vi "manipulator Controller.vi"(8 "error in":errorcluster) -> ()   [LabVIEW 2020]
doc: "This VI executes continuously carrying out the current operation and responding to updates or new operations. It will often contain the timing or control code that is difficult to place directly in TeleOp. This VI generally opens all sensors and motors and isolates the rest of the robot code from knowing how the operations are carried out."
uses:
  <vilib>/Rock Robotics/WPI/Framework/Completion Status.ctl
  manipulator Setpoints.ctl
  manipulator Operations.ctl
  Typedefs/Teleop Manipulator Commands.ctl
  Typedefs/Cube Shooting Presets.ctl
  <vilib>/Rock Robotics/WPI/ThirdParty/REV Robotics/REVLib/Typedef/Spark MAX Sensor Type.ctl
  <vilib>/Rock Robotics/WPI/ThirdParty/REV Robotics/REVLib/Typedef/Spark MAX Idle Mode.ctl
  <vilib>/Rock Robotics/WPI/ThirdParty/REV Robotics/REVLib/Typedef/Spark MAX Control Type.ctl
  Typedefs/Shoot Cube State.ctl
  782eae61-a325-4965-976c-c64f6a44d010.vi
  Framework/Robot Global Data.vi
  <vilib>/Rock Robotics/Network Tables/NT Write Boolean.vi
  <vilib>/ptbypt/NI_PtbyPt.lvlib
panel:
  out "Waveform Chart":cluster{u32, "mean":dbl}(graph)
  out "Abs Wrist Position":dbl
  in  "Interactive Values":T1={"Operation"=enum."Reserve", "Immediate Parameters"={"Wrist Power"=0.0, "Cascade Power"=0.0}, "Griddy Parameters"={"Griddy Command"=enum."idle", "Flip Wrist?"=FALSE}, "Reset Parameters"={"Reset Wrist"=FALSE, "Reset Cascade"=FALSE}, "Shoot Cube Parameters"={"Shot Preset"=enum."shoot mid"}}
  out "Current\nCmd":string
  in  "Buttons":cluster{"Execute Cmd":bool, "Abort Cmd":bool}
  out "Command Timing":cluster{"Start Time (ms)":u32, "Iterations":i32}
  out "Status":T5
  # "Tip: It may be helpful to observe inputs and sensor values.\nYou may also want to display tuning or debugging controls."
  # "Interactive Command: You may fill in the settings for a command\nand schedule it with the Execute button. You can observe and abort\nany command while fine tuning the code for the controller."
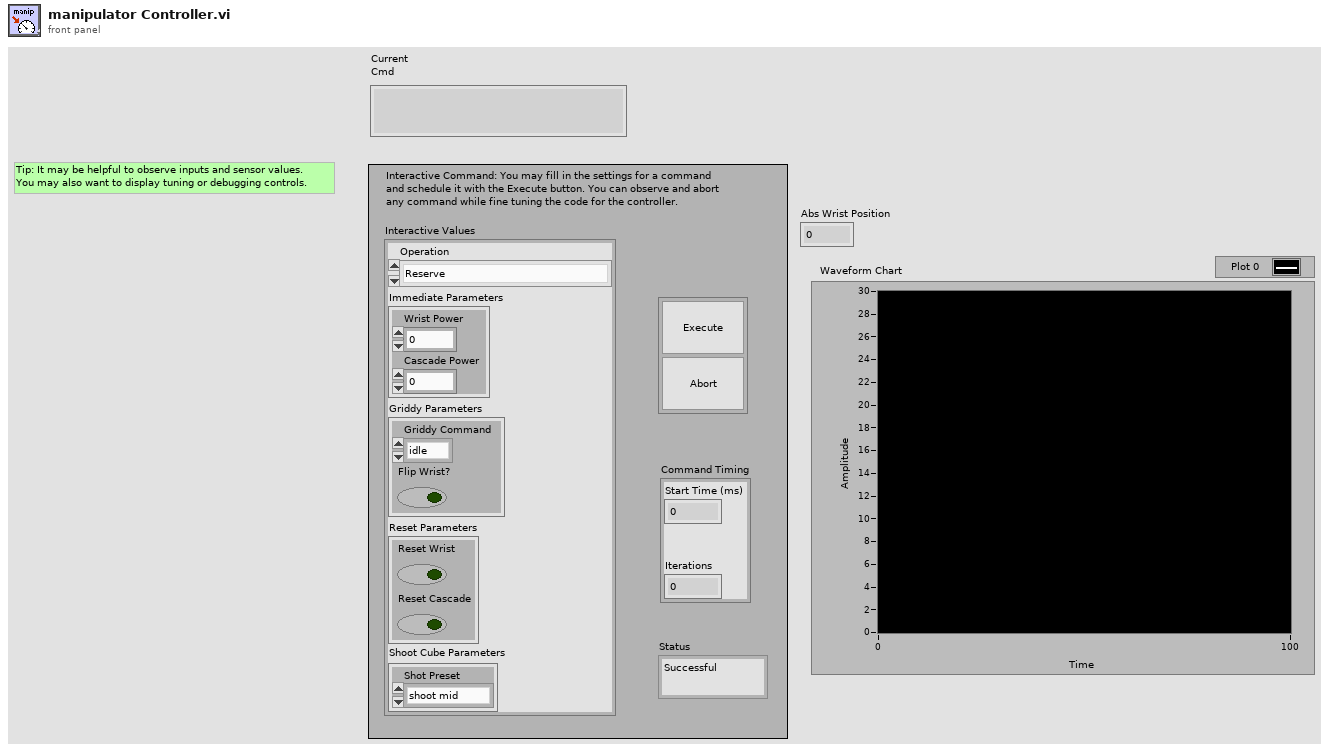
[diagram p1: front panel]
types:
  T1 = typedef "manipulator Setpoints.ctl" = cluster{"Operation":T2, "Immediate Parameters":cluster{"Wrist Power":dbl, "Cascade Power":dbl}, "Griddy Parameters":cluster{"Griddy Command":T3, "Flip Wrist?":bool}, "Reset Parameters":cluster{"Reset Wrist":bool, "Reset Cascade":bool}, "Shoot Cube Parameters":cluster{"Shot Preset":T4}}
  T2 = typedef "manipulator Operations.ctl" = enum16{"Reserve", "Read Current", "Immediate", "Reset Manipulator", "Grid-dy", "Shoot Cubes"}
  T3 = typedef "Teleop Manipulator Commands.ctl" = enum16{"idle", "intake cone sideways", "intake cone upright", "intake cone feeder", "intake cube feeder", "intake cube", "score low cone", "score low cube", "score mid cone", "score mid cube", "score high cone", "score high cube", "score mid cone up"}
  T4 = typedef "Cube Shooting Presets.ctl" = enum16{"shoot low", "shoot mid", "shoot high"}
  T5 = typedef "Completion Status.ctl" = enum16{"Successful", "Aborted", "Incomplete"}
  T6 = cluster{"P Gain":dbl, "I Gain":dbl, "D Gain":dbl, "F Gain":dbl, "I Zone":dbl, "Min Output":dbl, "Max Output":dbl}
  T7 = typedef "Spark MAX Idle Mode.ctl" = enum16{"Coast", "Brake"}
  T8 = typedef "Spark MAX Sensor Type.ctl" = enum16{"No Sensor", "Hall Sensor", "Encoder", "-Not Available-", "Analog", "Alternate Encoder", "Duty Cycle"}
  T9 = typedef "WPI_MotorControlDeviceRef.ctl" = cluster{"DeviceStatus":errorcluster, "Type":T10, "PWM":cluster{"PWM Channel":T11, "DeadBand":T12}, "CAN":cluster{"Device Number":u8, "SetOutput VI Ref":variant, "GetOutput VI Ref":variant, "Enable VI Ref":variant, "Disable VI Ref":variant, "Data":variant}, "Invert":bool, "DIO PWM":cluster{"PWM \"Enable\" Channel":T11, "DIOChannel":T13, "PWM Rate":dbl}}
  T10 = typedef "WPI_MotorControlType.ctl" = enum16{"PWM", "CAN", "DIO PWM"}
  T11 = typedef "FPGA_DIOPWMChannel.ctl" = enum8{"PWM 0", "PWM 1", "PWM 2", "PWM 3", "PWM 4", "PWM 5", "PWM 6", "PWM 7", "PWM 8", "PWM 9", "PWM MXP 0", "PWM MXP 1", "PWM MXP 2", "PWM MXP 3", "PWM MXP 4", "PWM MXP 5", "PWM MXP 6", "PWM MXP 7", "PWM MXP 8", "PWM MXP 9", "Invalid"}
  T12 = typedef "WPI_PWMDeadband.ctl" = cluster{"Name":string, "maxPositivePwm":i32, "minPositivePwm":i32, "centerPwm":i32, "maxNegativePwm":i32, "minNegativePwm":i32, "angularRange":u16}
  T13 = typedef "FPGA_DIOChannel.ctl" = enum8{"DIO 0", "DIO 1", "DIO 2", "DIO 3", "DIO 4", "DIO 5", "DIO 6", "DIO 7", "DIO 8", "DIO 9", "DIO MXP 0", "DIO MXP 1", "DIO MXP 2", "DIO MXP 3", "DIO MXP 4", "DIO MXP 5", "DIO MXP 6", "DIO MXP 7", "DIO MXP 8", "DIO MXP 9", "DIO MXP 10", "DIO MXP 11", "DIO MXP 12", "DIO MXP 13", "DIO MXP 14", "DIO MXP 15", "SPI Port CS1", "SPI Port CS2", "SPI Port CS3", "SPI Port MISO", "SPI Port MOSI", "Invalid"}
  T14 = typedef "Command Status Info.ctl" = cluster{"Name":string, "Status":T5, "notifier out":T15}
  T15 = typedef "Completion Notifier.ctl" = refnum<notifier>
  T16 = cluster{"Current Command":T1, "Command Timing":cluster{"Start Time (ms)":u32, "Iterations":i32}, "Command Arguments":cluster{"Command Info":T14, "Description":string, "Default Command":T1, "queue out":refnum<queue>, "Subsystem Name":string}}
  T17 = cluster{u32, "Immediate Parameters":cluster{"Wrist Power":dbl, "Cascade Power":dbl}}
  T18 = typedef "Spark MAX Control Type.ctl" = enum16{"Percent VBus", "Voltage", "Velocity", "Position", "Smart Motion", "Current", "Smart Velocity"}
  T19 = cluster{"Reset Wrist":bool, "Reset Cascade":bool}
  T20 = cluster{"Shot Config":cluster{"Wrist Prep Position":dbl, "Wrist Prep Margin":dbl, "Cascade Safety Position":dbl}, "Shot Parameters":cluster{"Shot Name":string, "Cascade Pow":dbl, "Shoot Position":dbl}[]}
  T21 = typedef "Shoot Cube State.ctl" = enum16{"Wrist Prep", "Shoot Cube", "Idle", "Finished"}
  T22 = cluster{"Wrist Prep Position":dbl, "Wrist Prep Margin":dbl, "Cascade Safety Position":dbl}
  T23 = cluster{"Shot Name":string, "Cascade Pow":dbl, "Shoot Position":dbl}[]
  T24 = cluster{"Shot Name":string, "Cascade Pow":dbl, "Shoot Position":dbl}
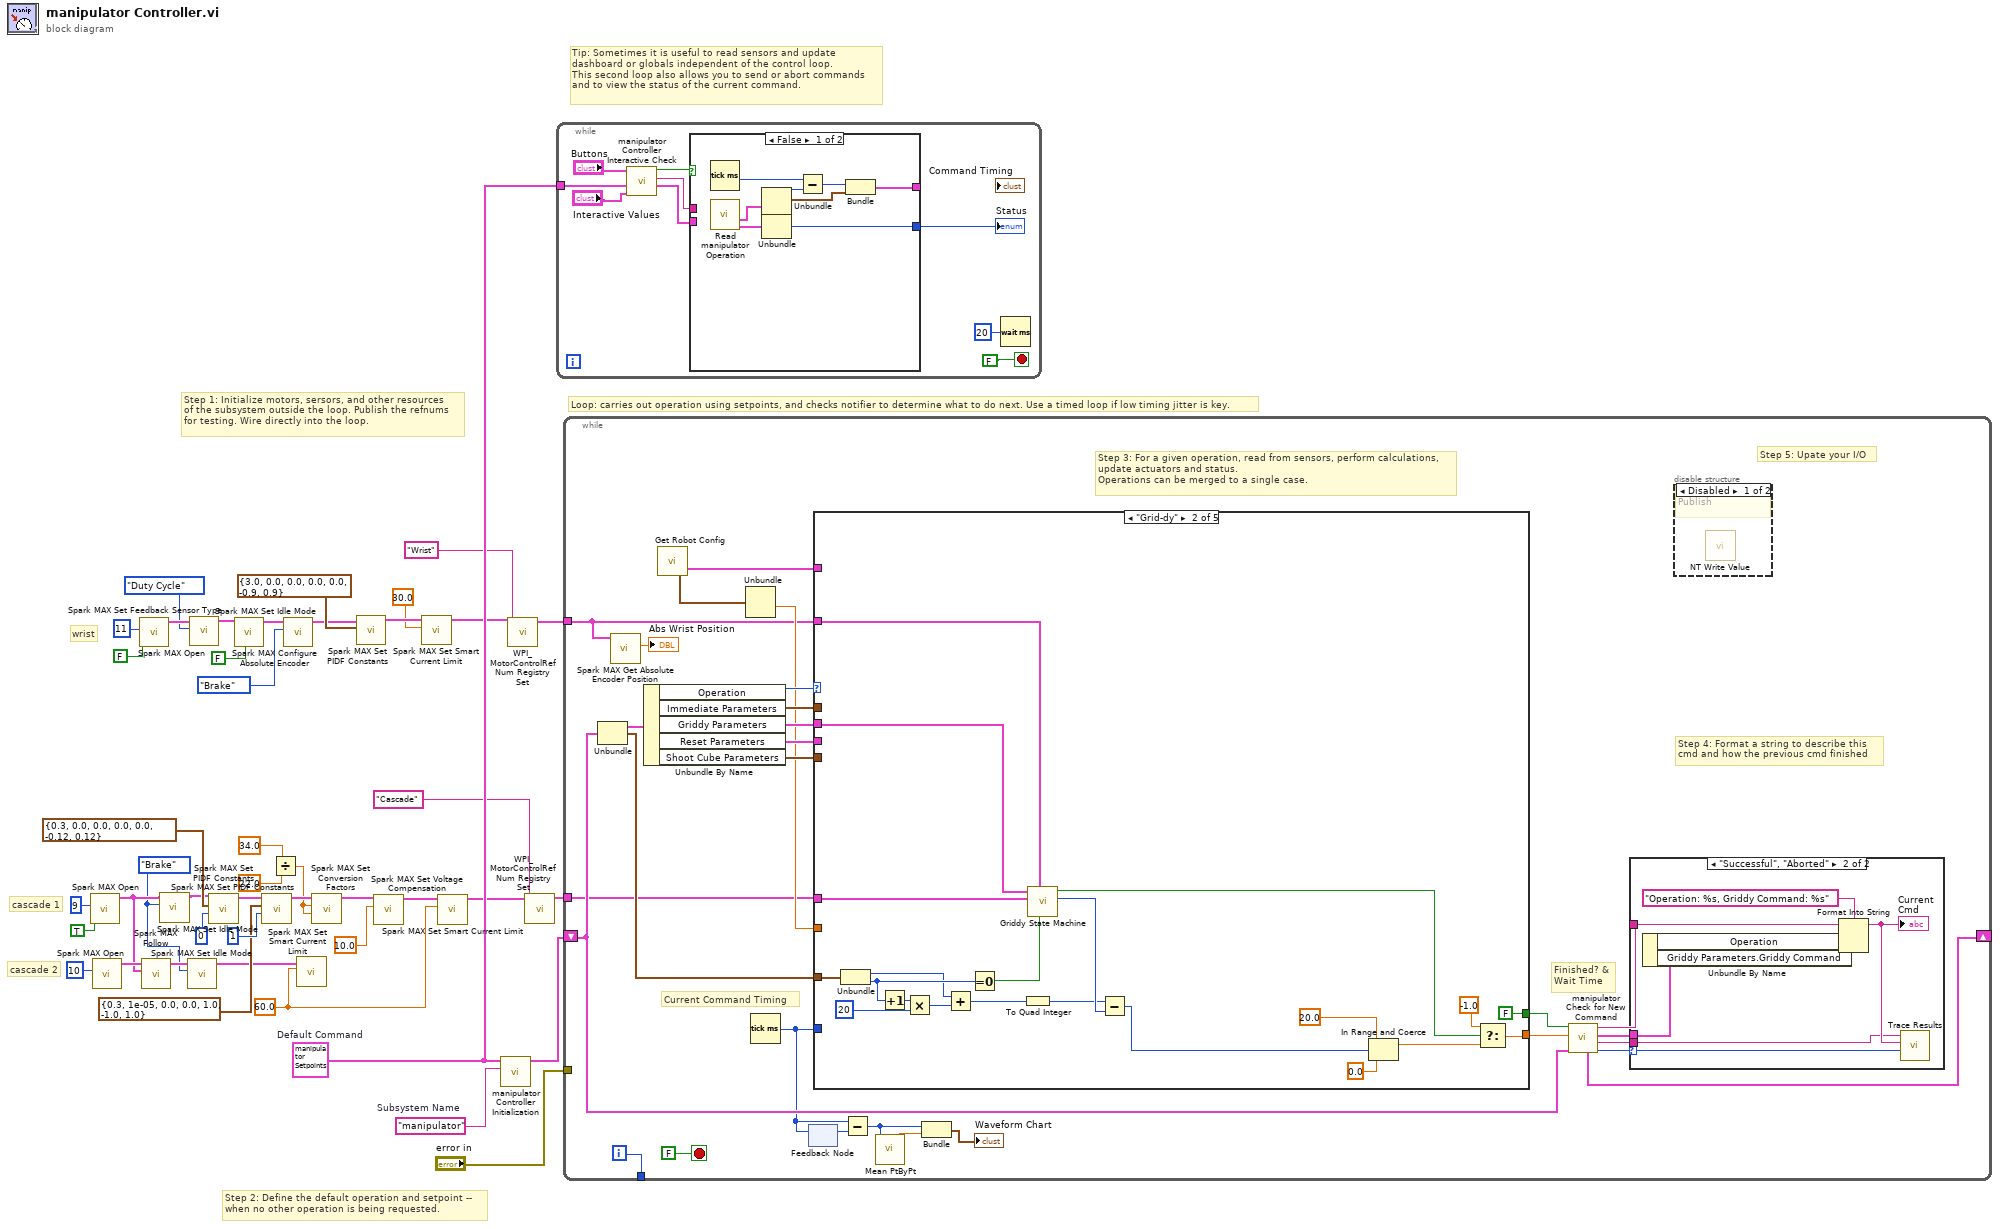
[diagram p0: block diagram]
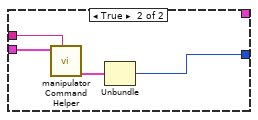
[diagram p2: hidden frame]
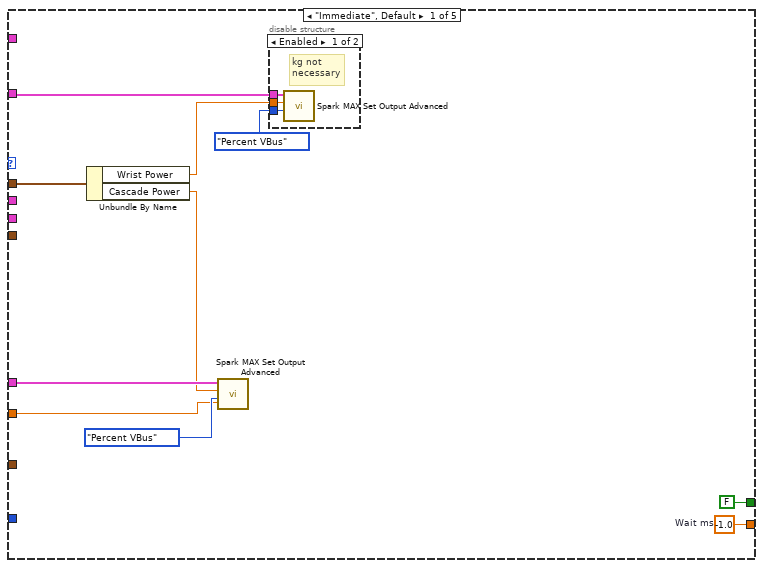
[diagram p3: hidden frame]
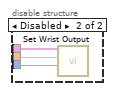
[diagram p4: hidden frame]
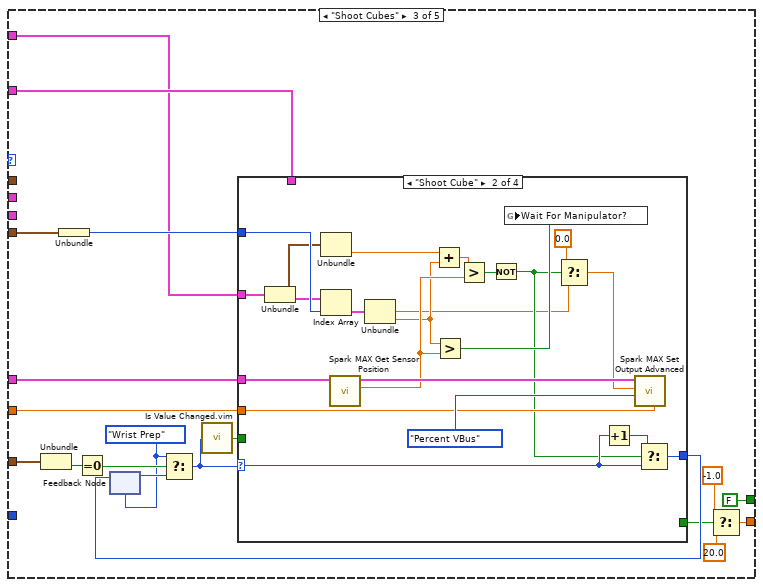
[diagram p5: hidden frame]
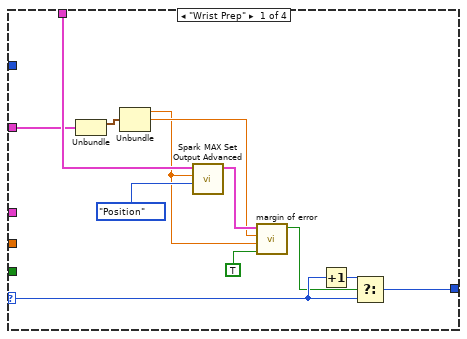
[diagram p6: hidden frame]
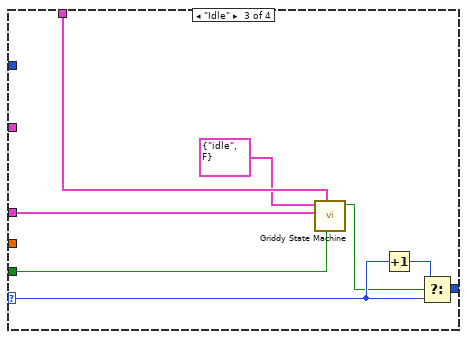
[diagram p7: hidden frame]
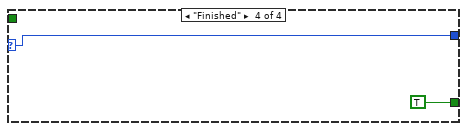
[diagram p8: hidden frame]
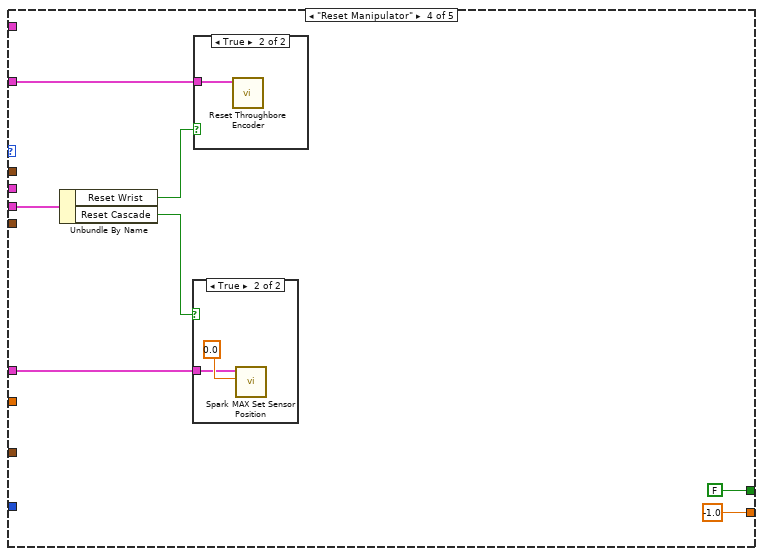
[diagram p9: hidden frame]
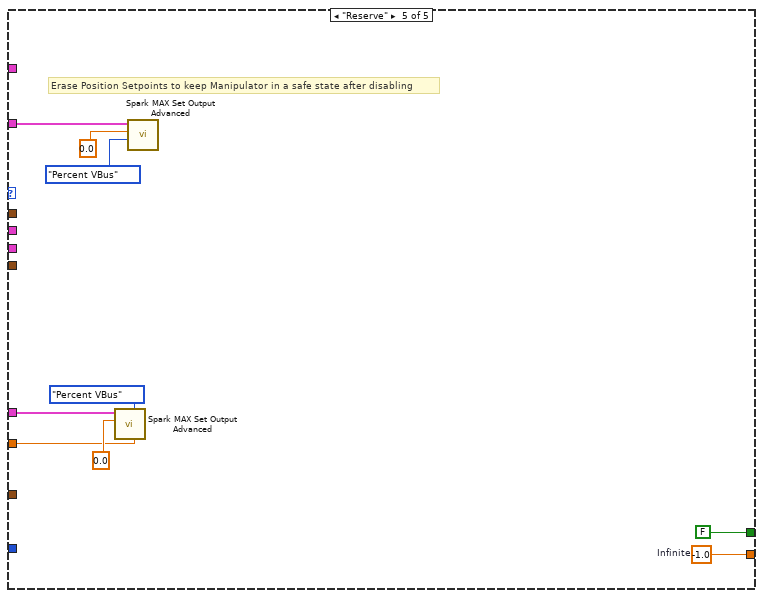
[diagram p12: hidden frame]
diagram:
  w1 = 60.0 ("Primay Current Limit (80A)")
  w15 = Spark_MAX_Idle_Mode."Brake" ("Idle Mode")
  w41 = T1 {"Operation"=enum."Reserve", "Immediate Parameters"={"Wrist Power"=0.0, "Cascade Power"=0.0}, "Griddy Parameters"={"Griddy Command"=enum."idle", "Flip Wrist?"=FALSE}, "Reset Parameters"={"Reset Wrist"=FALSE, "Reset Cascade"=FALSE}, "Shoot Cube Parameters"={"Shot Preset"=enum."shoot mid"}}  # Default Command
  w42 = "manipulator"  # Subsystem Name
  # "cascade 1"
  # "cascade 2"
  # "wrist"
  # "Tip: Sometimes it is useful to read sensors and update\ndashboard or globals independent of the control loop.\nThis second loop also allows you to send or abort commands\nand to view the status of the current command."
  # "Step 2: Define the default operation and setpoint --\nwhen no other operation is being requested."
  # "Step 1: Initialize motors, sersors, and other resources\nof the subsystem outside the loop. Publish the refnums\nfor testing. Wire directly into the loop."
  # "Loop: carries out operation using setpoints, and checks notifier to determine what to do next. Use a timed loop if low timing jitter is key."
  n1 = call <vilib>:"Spark MAX Open.vi"("Invert"=TRUE, "Device Number"=u8 9) -> ("MotorControlDeviceRef"=w35:T9)  [unwired: 8 in, 1 out]
  n2 = call <vilib>:"Spark MAX Open.vi"("Device Number"=u8 10) -> ("MotorControlDeviceRef"=w36:T9)  [unwired: 9 in, 1 out]
  n3 = call <vilib>:"Spark MAX Open.vi"("Invert"=FALSE, "Device Number"=u8 11) -> ("MotorControlDeviceRef"=w34:T9)  [unwired: 8 in, 1 out]
  n4 = call <vilib>:"Spark MAX Follow.vi"("Master Controller"=w35, "MotorControlDeviceRef"=w36) -> ("MotorControlDeviceRef"=w16:T9)  [unwired: 8 in, 1 out]
  n5 = call <vilib>:"Spark MAX Set Idle Mode.vi"("Idle Mode"=w15, "MotorControlDeviceRef in"=w35) -> ("MotorControlDeviceRef out"=w27:T9)  [unwired: 8 in, 1 out]
  n6 = call <vilib>:"Spark MAX Set Idle Mode.vi"("Idle Mode"=w15, "MotorControlDeviceRef in"=w16) -> ("MotorControlDeviceRef out"=w2:T9)  [unwired: 8 in, 1 out]
  n7 = call <vilib>:"Spark MAX Set Feedback Sensor Type.vi"("Sensor Type"=Spark_MAX_Sensor_Type."Duty Cycle", "MotorControlDevRef"=w34) -> ("MotorControlDeviceRef"=w32:T9)  [unwired: 8 in, 1 out]
  n8 = call <vilib>:"Spark MAX Set PIDF Constants.vi"("PIDF Slot"=0, "PID Constants"=T6 {"P Gain"=0.3, "I Gain"=0.0, "D Gain"=0.0, "F Gain"=0.0, "I Zone"=0.0, "Min Output"=-0.12, "Max Output"=0.12} ("cascade PID"), "MotorControlDeviceRef"=w27) -> ("MotorControlDeviceRef"=w14:T9)  [unwired: 7 in, 1 out]
  n9 = call <vilib>:"Spark MAX Configure Absolute Encoder.vi"("Inverted (F)"=FALSE, "MotorControlDeviceRef in"=w32) -> ("MotorControlDeviceRef out"=w26:T9)  [unwired: 8 in, 1 out]
  n10 = call <vilib>:"Spark MAX Set PIDF Constants.vi"("PIDF Slot"=1, "PID Constants"=T6 {"P Gain"=0.3, "I Gain"=1e-05, "D Gain"=0.0, "F Gain"=0.0, "I Zone"=1.0, "Min Output"=-1.0, "Max Output"=1.0}, "MotorControlDeviceRef"=w14) -> ("MotorControlDeviceRef"=w11:T9)  [unwired: 7 in, 1 out]
  n11 = Divide(x=34.0, y=22.0) -> (x/y=w5:dbl)
  n12 = call <vilib>:"Spark MAX Set Idle Mode.vi"("Idle Mode"=Spark_MAX_Idle_Mode."Brake", "MotorControlDeviceRef in"=w26) -> ("MotorControlDeviceRef out"=w25:T9)  [unwired: 8 in, 1 out]
  n13 = call <vilib>:"Spark MAX Set Smart Current Limit.vi"("Primay Current Limit (80A)"=w1, "MotorControlDeviceRef in"=w2) -> ()  [unwired: 8 in, 2 out]
  n14 = call <vilib>:"Spark MAX Set Conversion Factors.vi"("Velocity Factor (1)"=w5, "Position Factor (1)"=w5, "MotorControlDeviceRef in"=w11) -> ("MotorControlDeviceRef out"=w8:T9)  [unwired: 7 in, 1 out]
  n15 = call <vilib>:"Spark MAX Set PIDF Constants.vi"("PID Constants"=T6 {"P Gain"=3.0, "I Gain"=0.0, "D Gain"=0.0, "F Gain"=0.0, "I Zone"=0.0, "Min Output"=-0.9, "Max Output"=0.9} ("wrist PID"), "MotorControlDeviceRef"=w25) -> ("MotorControlDeviceRef"=w19:T9)  [unwired: 8 in, 1 out]
  n16 = call <vilib>:"Spark MAX Set Voltage Compensation.vi"("Nominal Voltage"=10.0, "MotorControlDeviceRef in"=w8) -> ("MotorControlDeviceRef out"=w4:T9)  [unwired: 8 in, 1 out]
  n17 = call <vilib>:"Spark MAX Set Smart Current Limit.vi"("Primay Current Limit (80A)"=30.0, "MotorControlDeviceRef in"=w19) -> ("MotorControlDeviceRef out"=w18:T9)  [unwired: 8 in, 1 out]
  n18 = call <vilib>:"Spark MAX Set Smart Current Limit.vi"("Primay Current Limit (80A)"=w1, "MotorControlDeviceRef in"=w4) -> ("MotorControlDeviceRef out"=w3:T9)  [unwired: 8 in, 1 out]
  n19 = call "manipulator Controller Initialization.vi"("Subsystem Name"=w42, "Default Command"=w41) -> ("Current Command"=w43:T16)  [unwired: 9 in]
  n20 = call <vilib>:"WPI_MotorControlRefNum Registry Set.vi"("refnum name"="Wrist", "MotorControlDevRef"=w18) -> ("MotorControlDevRef"=w23:T9)  [unwired: 8 in, 1 out]
  n21 = call <vilib>:"WPI_MotorControlRefNum Registry Set.vi"("refnum name"="Cascade", "MotorControlDevRef"=w3) -> ("MotorControlDevRef"=w21:T9)  [unwired: 8 in, 1 out]
  n22 = while {
    tunnel: w41 -> [w50]
    stop <- FALSE stop-if-true
    n23 = call "manipulator Controller Interactive Check.vi"("Interactive Command in"="Interactive Values", "Default Command"=w50, "Buttons"="Buttons") -> ("Interactive Command out"=w47:T1, "Trace String"=w48:string, "Schedule"=w49:bool)  [unwired: 6 in]
    n24 = case shown="False" w49 {
      tunnel: [w61 w65] -> w46
      tunnel: w47 -> [_ w63]
      tunnel: [w57 _] -> _
      tunnel: w48 -> [_ w64]
      frame False {
        n25 = Tick Count (ms)() -> (millisecond timer value=w56:u32)
        n26 = call "Read manipulator Operation.vi"() -> ("Command Info"=w54:T14, "SubSystem Data"=w55:T1)  [unwired: 9 in, 1 out]
        n27 = Unbundle(w55) -> ("Operation"=w60:T2, "Immediate Parameters"=w58:cluster{"Wrist Power":dbl, "Cascade Power":dbl})  [unwired: 3 out]
        n28 = Unbundle(w54) -> ("Status"=w61:T5)  [unwired: 2 out]
        n29 = Subtract(x=w56, y=w60) -> (x-y=w59:u32)
        n30 = Bundle(w59, "Immediate Parameters"=w58) -> (w57:T17)  [unwired: 1 in]
      }
      frame True {
        n31 = call "manipulator Command Helper.vi"("Description"=w64, "SubSystem Data"=w63) -> ("Command Info Out"=w62:T14)  [unwired: 7 in, 2 out]
        n32 = Unbundle(w62) -> ("Status"=w65:T5)  [unwired: 2 out]
      }
    }
    "Status" <- w46
    n33 = Wait (ms)(milliseconds to wait=u32 20) -> ()  [unwired: 1 out]
  }
  n34 = while {
    shift-right: [w87] -> _
    shift-left: w43 -> [w80]
    tunnel: [w92] -> _
    tunnel: "error in" -> [_]
    tunnel: w23 -> [w70]
    tunnel: w21 -> [w69]
    i -> [w92]
    stop <- FALSE stop-if-true
    # "Step 5: Upate your I/O"
    # "Step 4: Format a string to describe this\ncmd and how the previous cmd finished"
    # "Current Command Timing"
    # "Finished? &\nWait Time"
    # "Step 3: For a given operation, read from sensors, perform calculations,\nupdate actuators and status.\nOperations can be merged to a single case."
    n35 = Unbundle(w80) -> ("Current Command"=w91:T1, "Command Timing"=w88:cluster{"Start Time (ms)":u32, "Iterations":i32})  [unwired: 1 out]
    n36 = call <vilib>:"Spark MAX Get Absolute Encoder Position.vi"("MotorControlDeviceRef in"=w70) -> ("Position"=→"Abs Wrist Position":dbl)  [unwired: 7 in, 3 out]
    n37 = Unbundle By Name(w91) -> ("Operation"=w90:T2, "Immediate Parameters"=w89:cluster{"Wrist Power":dbl, "Cascade Power":dbl}, "Griddy Parameters"=w79:cluster{"Griddy Command":T3, "Flip Wrist?":bool}, "Reset Parameters"=w78:T19, "Shoot Cube Parameters"=w77:cluster{"Shot Preset":T4})
    n38 = call "Get Robot Config.vi"() -> ("Cascade FeedForward Constants"=w75:cluster{"kA":dbl, "kS":dbl, "kG":dbl, "kV":dbl}, "Shoot Cube Config"=w76:T20)  [unwired: 12 in, 6 out]
    n39 = Unbundle(w75) -> ("kG"=w74:dbl)  [unwired: 3 out]
    n40 = Tick Count (ms)() -> (millisecond timer value=w72:u32)
    n41 = feedback-in #1(w72) -> ()
    n42 = feedback #1() -> (w73:u32)  [unwired: 1 in]
    n43 = case shown="\"Grid-dy\"" w90 {
      tunnel: [w103 w127 w137 -1.0 ("Infinite") w212] -> w85
      tunnel: [FALSE ("ignore previous (F)") FALSE ("ignore previous (F)") FALSE ("ignore previous (F)") FALSE ("ignore previous (F)") FALSE ("ignore previous (F)")] -> w86
      tunnel: w88 -> [_ w119 w149 _ _]
      tunnel: w89 -> [w99 _ _ _ _]
      tunnel: w72 -> [_ _ _ _ _]
      tunnel: w79 -> [_ w124 _ _ _]
      tunnel: w70 -> [w101 w128 w143 w194 w208]
      tunnel: w78 -> [_ _ _ w198 _]
      tunnel: w69 -> [w97 w130 w142 w195 w206]
      tunnel: w77 -> [_ _ w141 _ _]
      tunnel: w76 -> [_ _ w132 _ _]
      tunnel: w74 -> [w94 _ w131 _ w204]
      frame "Immediate", Default {
        w103 = -1.0  # Wait ms
        n44 = Unbundle By Name(w99) -> ("Wrist Power"=w98:dbl, "Cascade Power"=w96:dbl)
        n45 = call <vilib>:"Spark MAX Set Output Advanced.vi"("Arbitrary Feed Forward (0)"=w94, "Control Mode"=Spark_MAX_Control_Type."Percent VBus", "Setpoint"=w96, "MotorControlDevRef"=w97) -> ()  [unwired: 6 in, 2 out]
        n46 = disable-structure shown="Enabled" {
          disable-tunnel: Spark_MAX_Control_Type."Percent VBus" ("Control Mode") -> [w106 w107]
          disable-tunnel: w101 -> [w105 w109]
          disable-tunnel: w98 -> [w104 w108]
          frame Enabled {
            # "kg not\nnecessary"
            n47 = call <vilib>:"Spark MAX Set Output Advanced.vi"("Control Mode"=w106, "Setpoint"=w104, "MotorControlDevRef"=w105) -> ()  [unwired: 7 in, 2 out]
          }
          frame Disabled {
            n48 = call "Set Wrist Output.vi"("Control Mode"=w107, "Setpoint"=w108, "MotorControlDevRef"=w109) -> ()  [unwired: 9 in]
          }
        }
      }
      frame "Grid-dy" {
        n49 = Unbundle(w119) -> ("Start Time (ms)"=w113:u32, "Iterations"=w115:i32)
        n50 = Increment(x=w115) -> (x+1=w116:i32)
        n51 = Multiply(x=w116, y=20) -> (x*y=w117:i32)
        n52 = Add(x=w113, y=w117) -> (x+y=w110:u32)
        n53 = Equal To 0?(x=w115) -> (x = 0?=w129:bool)
        n54 = To Quad Integer(1:w110) -> (0:w111:i64)
        n55 = call "Griddy State Machine.vi"("Griddy Started?"=w129, "Wrist"=w128, "Cascade"=w130, "Griddy Parameters"=w124) -> ("Current Time"=w114:u32, "Is Finished?"=w123:bool)  [unwired: 6 in]
        n56 = Subtract(x=w111, y=w114) -> (x-y=w112:i64)
        n57 = In Range and Coerce(upper limit=20.0 ("Infinite"), x=w112, lower limit=0.0) -> (coerced(x)=w120:dbl)  [unwired: 1 out]
        n58 = Select(t=-1.0 ("f"), s=w123, f=w120) -> (s? t:f=w127:dbl)
      }
      frame "Shoot Cubes" {
        w144 = Shoot_Cube_State."Wrist Prep"
        n59 = Unbundle(w149) -> ("Iterations"=w148:i32)  [unwired: 1 out]
        n60 = Unbundle(w141) -> ("Shot Preset"=w140:T4)
        n61 = Equal To 0?(x=w148) -> (x = 0?=w146:bool)
        n62 = feedback #2(w144) -> (w147:T21)
        n63 = Select(t=w144, s=w146, f=w147) -> (s? t:f=w139:T21)
        n64 = call "Is Value Changed.vim"("value"=w139) -> ("changed or first call?"=w138:bool)
        n65 = case shown="\"Shoot Cube\"" w139 {
          selector: w139 -> [w154 w176 w189 w193]
          tunnel: [w156 w178 w191 w193] -> w145
          tunnel: w143 -> [w161 _ w187 _]
          tunnel: w132 -> [w160 w183 _ _]
          tunnel: w142 -> [_ w175 w184 _]
          tunnel: w140 -> [_ w182 _ _]
          tunnel: w131 -> [_ w179 _ _]
          tunnel: w138 -> [_ _ w185 _]
          tunnel: [_ _ _ TRUE ("ignore previous (F)")] -> w136
          frame "Wrist Prep" {
            n66 = Unbundle(w160) -> ("Shot Config"=w152:T22)  [unwired: 1 out]
            n67 = Unbundle(w152) -> ("Wrist Prep Position"=w150:dbl, "Wrist Prep Margin"=w151:dbl)  [unwired: 1 out]
            n68 = call <vilib>:"Spark MAX Set Output Advanced.vi"("Control Mode"=Spark_MAX_Control_Type."Position", "Setpoint"=w150, "MotorControlDevRef"=w161) -> ("MotorControlDevRef"=w157:T9)  [unwired: 7 in, 1 out]
            n69 = call "margin of error.vi"("Wrist Motor?"=TRUE, "setpoint"=w150, "margin of error"=w151, "Motor In"=w157) -> ("In Range?"=w153:bool)  [unwired: 6 in, 1 out]
            n70 = Increment(x=w154) -> (x+1=w155:T21)
            n71 = Select(t=w155, s=w153, f=w154) -> (s? t:f=w156:T21)
          }
          frame "Shoot Cube" {
            n72 = Unbundle(w183) -> ("Shot Config"=w172:T22, "Shot Parameters"=w173:T23)
            n73 = Unbundle(w172) -> ("Cascade Safety Position"=w166:dbl)  [unwired: 2 out]
            n74 = Index Array(array=w173, index=w182) -> (element=w181:T24)
            n75 = call <vilib>:"Spark MAX Get Sensor Position.vi"("MotorControlDevRef in"=w175) -> ("Sensor Position"=w171:dbl, "MotorControlDevRef out"=w174:T9)  [unwired: 7 in, 2 out]
            n76 = Unbundle(w181) -> ("Cascade Pow"=w164:dbl, "Shoot Position"=w168:dbl)  [unwired: 1 out]
            n77 = Add(x=w166, y=w168) -> (x+y=w167:dbl)
            n78 = Greater?(x=w168, y=w171) -> (0:w169:bool)
            n79 = Greater?(x=w167, y=w171) -> (0:w170:bool)
            n80 = Not(x=w170) -> (.not. x?=w165:bool)
            n81 = global write "Robot Global Data.vi" "Wait For Manipulator?"(w169) -> ()
            n82 = Select(t=0.0 ("f"), s=w165, f=w164) -> (s? t:f=w162:dbl)
            n83 = Increment(x=w176) -> (x+1=w177:T21)
            n84 = call <vilib>:"Spark MAX Set Output Advanced.vi"("Arbitrary Feed Forward (0)"=w179, "Control Mode"=Spark_MAX_Control_Type."Percent VBus", "Setpoint"=w162, "MotorControlDevRef"=w174) -> ()  [unwired: 6 in, 2 out]
            n85 = Select(t=w177, s=w165, f=w176) -> (s? t:f=w178:T21)
          }
          frame "Idle" {
            n86 = call "Griddy State Machine.vi"("Griddy Started?"=w185, "Wrist"=w187, "Cascade"=w184, "Griddy Parameters"=cluster{"Griddy Command":T3, "Flip Wrist?":bool} {"Griddy Command"=enum."idle", "Flip Wrist?"=FALSE}) -> ("Is Finished?"=w188:bool)  [unwired: 6 in, 1 out]
            n87 = Increment(x=w189) -> (x+1=w190:T21)
            n88 = Select(t=w190, s=w188, f=w189) -> (s? t:f=w191:T21)
          }
          frame "Finished" {
          }
        }
        n89 = feedback-in #2(w145) -> ()
        n90 = Select(t=-1.0, s=w136, f=20.0) -> (s? t:f=w137:dbl)
      }
      frame "Reset Manipulator" {
        n91 = Unbundle By Name(w198) -> ("Reset Wrist"=w196:bool, "Reset Cascade"=w197:bool)
        n92 = case shown="True" w197 {
          tunnel: w195 -> [_ w201]
          frame False {
          }
          frame True {
            n93 = call <vilib>:"Spark MAX Set Sensor Position.vi"("Position"=0.0 ("Setpoint"), "MotorControlDeviceRef"=w201) -> ()  [unwired: 8 in, 2 out]
          }
        }
        n94 = case shown="True" w196 {
          tunnel: w194 -> [_ w203]
          frame False {
          }
          frame True {
            n95 = call "Reset Throughbore Encoder.vi"("MotorControlDeviceRef in"=w203) -> ()  [unwired: 10 in, 1 out]
          }
        }
      }
      frame "Reserve" {
        w212 = -1.0  # Infinite
        # "Erase Position Setpoints to keep Manipulator in a safe state after disabling"
        n96 = call <vilib>:"Spark MAX Set Output Advanced.vi"("Arbitrary Feed Forward (0)"=w204, "Control Mode"=Spark_MAX_Control_Type."Percent VBus", "Setpoint"=0.0, "MotorControlDevRef"=w206) -> ()  [unwired: 6 in, 2 out]
        n97 = call <vilib>:"Spark MAX Set Output Advanced.vi"("Control Mode"=Spark_MAX_Control_Type."Percent VBus", "Setpoint"=0.0, "MotorControlDevRef"=w208) -> ()  [unwired: 7 in, 2 out]
      }
    }
    n98 = Subtract(x=w72, y=w73) -> (x-y=w67:u32)
    n99 = call <vilib>:"Mean PtByPt.vi"("x"=w67) -> ("mean"=w68:dbl)  [unwired: 3 in, 1 out]
    n100 = Bundle(w67, "mean"=w68) -> (→"Waveform Chart":cluster{u32, "mean":dbl})  [unwired: 1 in]
    n101 = call "manipulator Check for New Command.vi"("Current Command"=w80, "Wait time (ms)"=w85, "Finished?"=w86) -> ("Completion"=w81:T5, "Subsystem Name"=w82:string, "Current Command"=w83:T1, "Initial Trace String"=w84:string, "NextCommand"=w87:T16)  [unwired: 4 in]
    n102 = case shown="\"Successful\", \"Aborted\"" w81 {
      selector: w81 -> [_ w220]
      tunnel: w84 -> [_ w216]
      tunnel: w83 -> [_ w217]
      tunnel: w82 -> [_ w213]
      frame "Incomplete", Default {
        # "Continuing current command"
      }
      frame "Successful", "Aborted" {
        # "Report and setup for next command"
        n103 = Unbundle By Name(w217) -> ("Operation"=w219:T2, "Griddy Parameters.Griddy Command"=w214:T3)
        n104 = Format Into String(format string="Operation: %s, Griddy Command: %s", initial string=w216, w219, w214) -> (resulting string=w215:string)  [unwired: 1 in, 1 out]
        "Current\nCmd" <- w215
        n105 = call <vilib>:"Trace Results.vi"("Status of previous command"=w220, "Description"=w215, "Subsystem"=w213) -> ()  [unwired: 9 in]
      }
    }
    n106 = disable-structure shown="Disabled" {
      frame Disabled {
        # "Publish"
        n107 = call-poly <vilib>:"NT Write Value.vi"() -> ()  [unwired: 11 in, 1 out]
      }
      frame Enabled {
      }
    }
  }
